vi "formatnnmsg.vi"(8 "error in (no error)":errorcluster, 9 "Numeric in":dbl, 10 "Numeric":i32, 11 "Boolean":bool) -> (0 "error out":errorcluster, 3 "String":string)   [LabVIEW 2018, in "nn.lvlib"]
uses:
  nn.lvlib
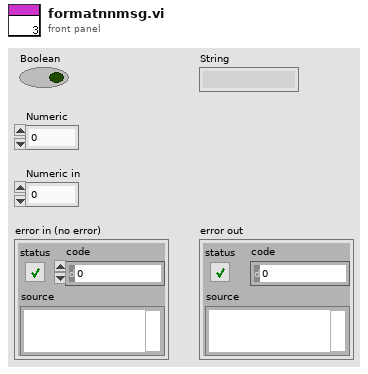
[diagram p1: front panel]
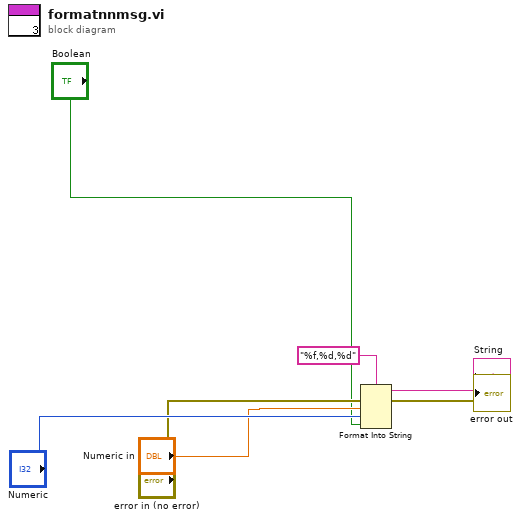
[diagram p0: block diagram]
diagram:
  n1 = Format Into String(format string="%f,%d,%d", error in="error in (no error)", "Numeric in", "Numeric", "Boolean") -> (resulting string=→"String":string, error out=→"error out":errorcluster)  [unwired: 1 in]
